vi "_RT Open Preference File.vi"() -> (0 "error":errorcluster, 3 "refnum":T1)   [LabVIEW 2012]
uses:
  <vilib>/Utility/config.llb/Config Data RefNum.ctl
  <vilib>/Utility/config.llb/NI_LVConfig.lvlib
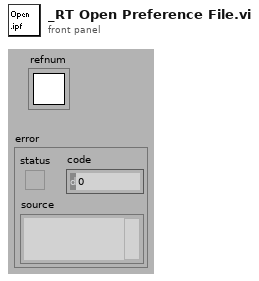
[diagram p1: front panel]
types:
  T1 = typedef "NI_LVConfig.lvlib/Config Data RefNum.ctl" = refnum<k1>
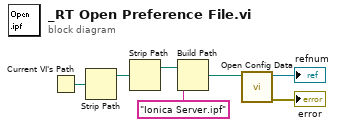
[diagram p0: block diagram]
diagram:
  n1 = Current VI's Path() -> (path=w1:path)
  n2 = Strip Path(path=w1) -> (stripped path=w2:path)  [unwired: 1 out]
  n3 = Strip Path(path=w2) -> (stripped path=w3:path)  [unwired: 1 out]
  n4 = Build Path(base path=w3, name or relative path="Ionica Server.ipf") -> (appended path=w4:path)
  n5 = call <vilib>:"Open Config Data.vi"("configuration file path"=w4) -> ("error out"=→"error":errorcluster, "refnum"=→"refnum":T1)  [unwired: 8 in, 1 out]
